vi "编译图形.vi"(8 "error in (no error)":errorcluster caption="错误输入（无错误）", 11 "程序 输入":refnum<class "程序.lvclass">) -> (0 "error out":errorcluster caption="错误输出", 3 "程序 输出":refnum<class "程序.lvclass">)   [LabVIEW 2018, in "程序.lvclass"]
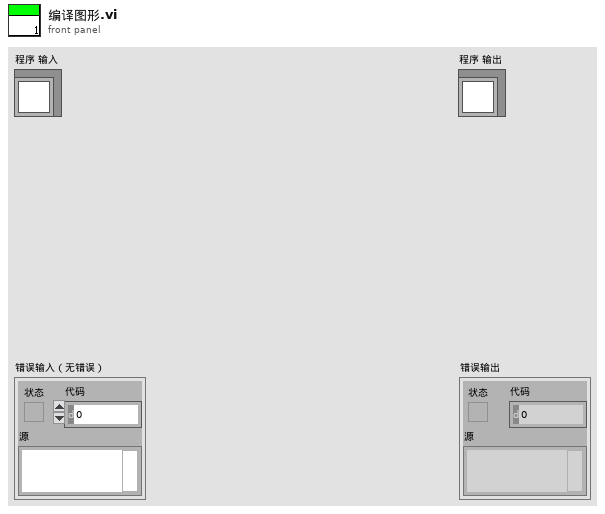
[diagram p1: front panel]
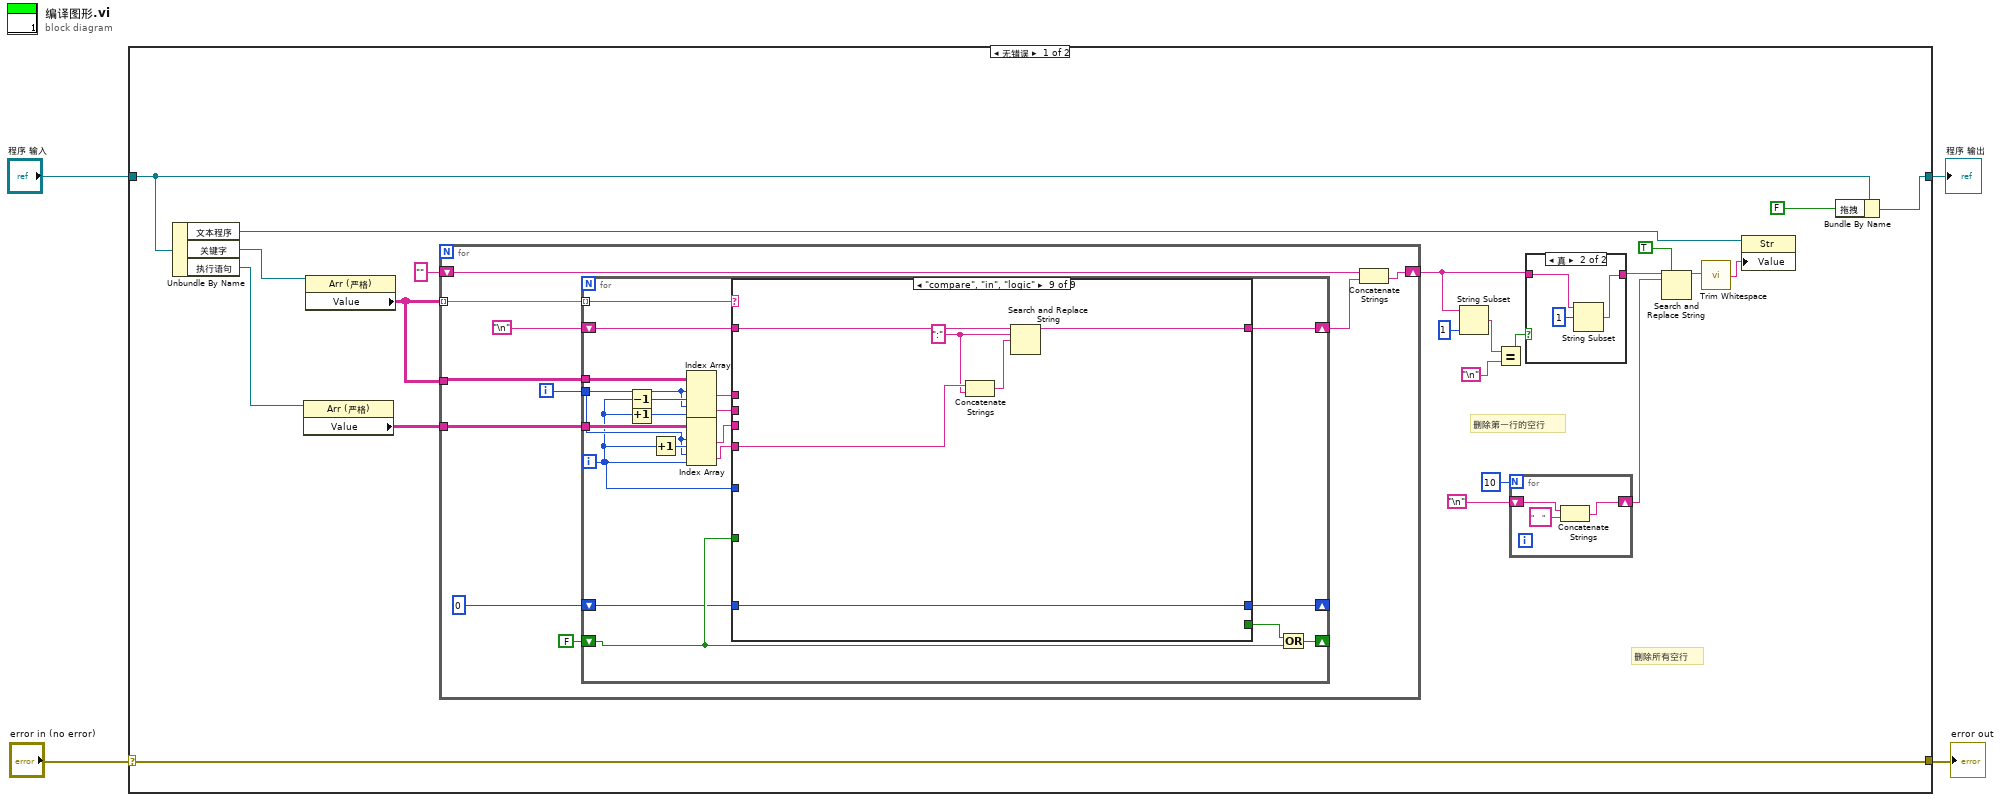
[diagram p0: block diagram]
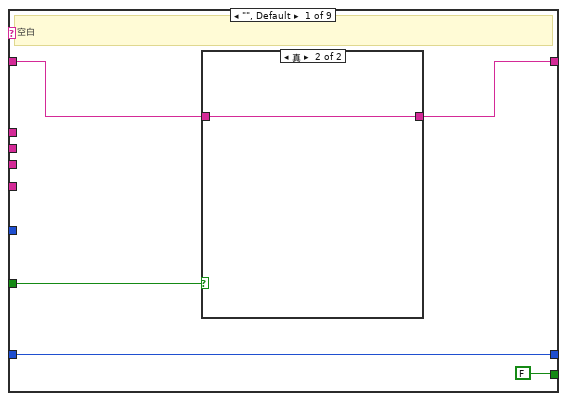
[diagram p3: hidden frame]
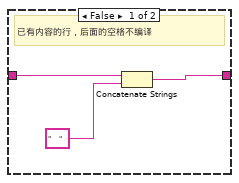
[diagram p4: hidden frame]
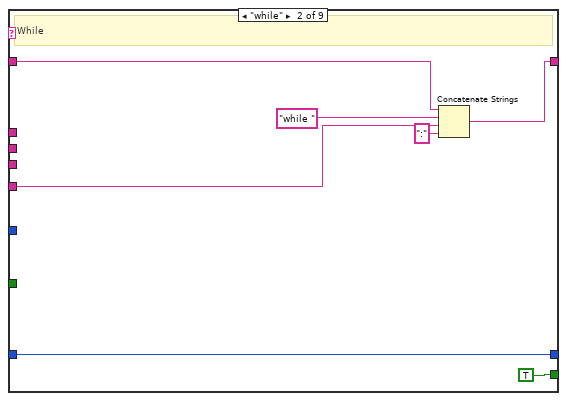
[diagram p5: hidden frame]
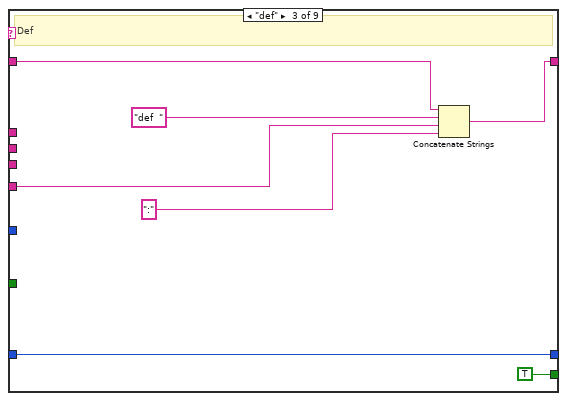
[diagram p6: hidden frame]
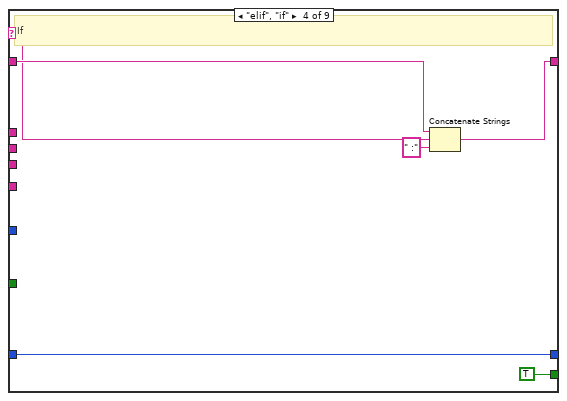
[diagram p7: hidden frame]
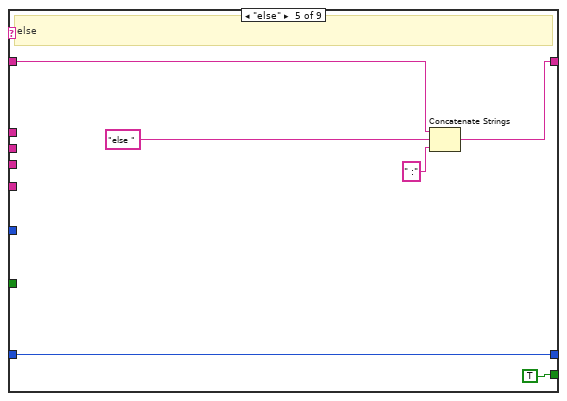
[diagram p8: hidden frame]
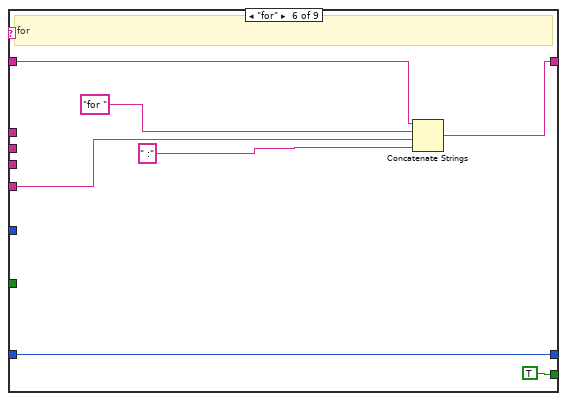
[diagram p9: hidden frame]
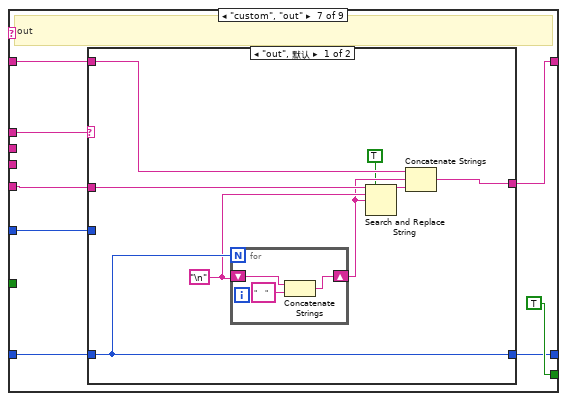
[diagram p10: hidden frame]
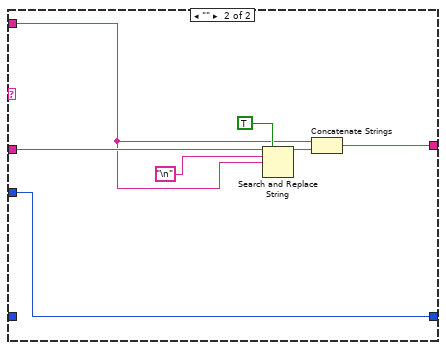
[diagram p11: hidden frame]
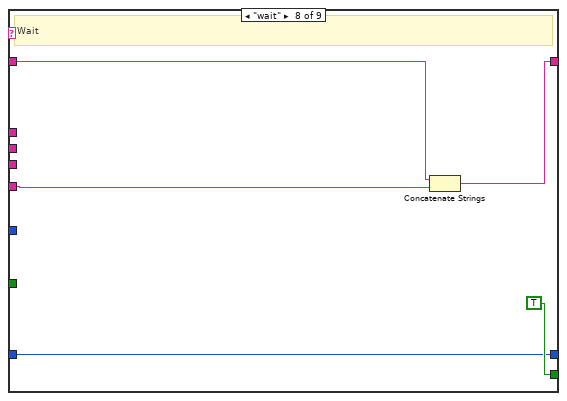
[diagram p12: hidden frame]
diagram:
  n1 = case shown="无错误" "error in (no error)" {
    selector: "error in (no error)" -> [w26 w143]
    tunnel: [w26 w143] -> w3
    tunnel: [w5 w142] -> w1
    tunnel: "程序 输入" -> [w7 w142]
    frame No Error {
      # "删除所有空行"
      # "删除第一行的空行"
      n2 = Unbundle By Name(w7) -> ("文本程序"=w20:refnum<vi>, "关键字"=w22:refnum<vi>, "执行语句"=w21:refnum<vi>)
      n3 = property class="Arr (严格)"(reference=w21) -> ("Value"=w23:string[][])  [unwired: 1 in, 2 out]
      n4 = property class="Arr (严格)"(reference=w22) -> ("Value"=w24:string[][])  [unwired: 1 in, 2 out]
      n5 = for {
        tunnel: w24 -> [w43] mode=indexing
        tunnel: w23 -> [w42]
        shift-right: [w38] -> w16
        shift-left: "" -> [w39]
        tunnel: w24 -> [w41]
        i -> [w40]
        n6 = for {
          tunnel: w43 -> [w62] mode=indexing
          shift-right: [w58] -> w37
          shift-left: "\n" -> [w56]
          tunnel: w42 -> [w60]
          tunnel: w41 -> [w55]
          tunnel: w40 -> [w52]
          shift-right: [w48] -> _
          shift-left: FALSE -> [w46]
          shift-right: [w45] -> _
          shift-left: 0 -> [w44]
          i -> [w51]
          n7 = Decrement(x=w51) -> (x-1=w54:i32)
          n8 = Increment(x=w51) -> (x+1=w50:i32)
          n9 = Increment(x=w51) -> (x+1=w57:i32)
          n10 = Index Array(array=w55, index (row) #1=w52, index (col) #1=w54, index (row) #2=w52, index (col) #2=w50) -> (element #1=w53:string, element #2=w49:string)
          n11 = Index Array(array=w60, index (row) #1=w52, index (col) #1=w57, index (row) #2=w52, index (col) #2=w51) -> (element #1=w61:string, element #2=w59:string)
          n12 = case shown="\"compare\", \"in\", \"logic\"" w62 {
            selector: w62 -> [_ _ _ w87 _ _ _ _ _]
            tunnel: [w67 w76 w83 w90 w94 w100 w110 w133 w136] -> w58
            tunnel: w61 -> [_ _ _ _ _ _ _ _ _]
            tunnel: w59 -> [_ w74 w82 _ _ w103 w112 w135 w139]
            tunnel: w56 -> [w66 w77 w84 w91 w95 w101 w111 w134 w140]
            tunnel: w53 -> [_ _ _ _ _ _ w109 _ _]
            tunnel: w51 -> [_ _ _ _ _ _ w108 _ _]
            tunnel: w49 -> [_ _ _ _ _ _ _ _ _]
            tunnel: [FALSE TRUE TRUE TRUE TRUE TRUE TRUE TRUE _] -> w47
            tunnel: w46 -> [w64 _ _ _ _ _ _ _ _]
            tunnel: [w63 w72 w79 w88 w92 w98 w106 w131 w141] -> w45
            tunnel: w44 -> [w63 w72 w79 w88 w92 w98 w105 w131 w141]
            frame "", Default {
              # "空白"
              n13 = case shown="真" w64 {
                tunnel: [w70 w71] -> w67
                tunnel: w66 -> [w69 w71]
                frame False {
                  # "已有内容的行，后面的空格不编译"
                  n14 = Concatenate Strings(w69, "    " ("字符串")) -> (w70:string)
                }
                frame True {
                }
              }
            }
            frame "while" {
              # "While"
              n15 = Concatenate Strings(w77, "while " ("字符串"), w74, ":" ("字符串")) -> (w76:string)
            }
            frame "def" {
              # "Def"
              n16 = Concatenate Strings(w84, "def  " ("字符串"), w82, ":" ("字符串")) -> (w83:string)
            }
            frame "elif", "if" {
              # "If"
              n17 = Concatenate Strings(w91, w87, " :" ("字符串")) -> (w90:string)
            }
            frame "else" {
              # "else"
              n18 = Concatenate Strings(w95, "else ", " :" ("字符串")) -> (w94:string)
            }
            frame "for" {
              # "for"
              n19 = Concatenate Strings(w101, "for " ("字符串"), w103, " :" ("字符串")) -> (w100:string)
            }
            frame "custom", "out" {
              # "out"
              n20 = case shown="\"out\", 默认" w109 {
                tunnel: w112 -> [w118 w126]
                tunnel: w111 -> [w120 w124]
                tunnel: [w119 w125] -> w110
                tunnel: w108 -> [_ w130]
                tunnel: [w117 w130] -> w106
                tunnel: w105 -> [w117 _]
                frame "out", Default {
                  w116 = "\n"
                  n21 = for {
                    N: w117 -> [_]
                    shift-right: [w122] -> w114
                    shift-left: w116 -> [w123]
                    n22 = Concatenate Strings(w123, "    " ("字符串")) -> (w122:string)
                  }
                  n23 = Search and Replace String(replace all?=TRUE ("替换全部？(F)"), input string=w118, search string=w116, replace string=w114) -> (result string=w115:string)  [unwired: 4 in, 3 out]
                  n24 = Concatenate Strings(w120, w114, w115) -> (w119:string)
                }
                frame "" {
                  n25 = Search and Replace String(replace all?=TRUE ("替换全部？(F)"), input string=w126, search string="\n", replace string=w124) -> (result string=w128:string)  [unwired: 4 in, 3 out]
                  n26 = Concatenate Strings(w124, w128) -> (w125:string)
                }
              }
            }
            frame "wait" {
              # "Wait"
              n27 = Concatenate Strings(w134, w135) -> (w133:string)
            }
            frame "compare", "in", "logic" {
              w138 = ":" ("搜索字符串")
              n28 = Concatenate Strings(w139, w138) -> (w137:string)
              n29 = Search and Replace String(input string=w140, search string=w138, replace string=w137) -> (result string=w136:string)  [unwired: 5 in, 3 out]
            }
          }
          n30 = Or(x=w47, y=w46) -> (x .or. y?=w48:bool)
        }
        n31 = Concatenate Strings(w39, w37) -> (w38:string)
      }
      n32 = String Subset(string=w16, length (rest)=1 ("长度（剩余）")) -> (substring=w18:string)  [unwired: 1 in]
      n33 = Equal?(x=w18, y="\n") -> (x = y?=w15:bool)
      n34 = for {
        N: 10 -> [_]
        shift-right: [w28] -> w11
        shift-left: "\n" -> [w29]
        n35 = Concatenate Strings(w29, "    " ("字符串")) -> (w28:string)
      }
      n36 = case shown="真" w15 {
        tunnel: w16 -> [w30 w33]
        tunnel: [w30 w31] -> w14
        frame False {
        }
        frame True {
          n37 = String Subset(string=w33, offset (0)=1 ("偏移量(0)")) -> (substring=w31:string)  [unwired: 1 in]
        }
      }
      n38 = Search and Replace String(replace all?=TRUE ("替换全部？(F)"), input string=w14, search string=w11) -> (result string=w9:string)  [unwired: 5 in, 3 out]
      n39 = call <vilib>:"Trim Whitespace.vi"("string"=w9) -> ("trimmed string"=w8:string)  [unwired: 1 in]
      n40 = property class="Str"(reference=w20, "Value"=w8) -> ()  [unwired: 1 in, 2 out]
      n41 = Bundle By Name(cluster=w7, "拖拽"=FALSE) -> (w5:refnum<class "程序.lvclass">)
    }
    frame Error {
    }
  }
  "error out" <- w3
  "程序 输出" <- w1
